vi "sitios sound.vi"() -> ()   [LabVIEW 2010]
uses:
  <vilib>/addons/PixeLINK/Low Level Functions/CAMERA_FEATURES.llb/TDPU-CameraFeatures-PixelFormat.ctl
  <vilib>/sound2/lvsound2.llb/Sound Data Format.ctl
  <vilib>/sound2/lvsound2.llb/Sound Output Task ID.ctl
  <vilib>/Utility/error.llb/DialogType.ctl
  <vilib>/Utility/file.llb/Write To Spreadsheet File (DBL).vi
  <vilib>/vision/NI_Vision_Development_Module.lvlib
panel:
  in  "Paso inicial":dbl=0.25
  out "Numeric":dbl
  out "output string":string
  in  "Sound Controls":T2={"device ID"=0, "sound format"={"sample rate (S/s)"=44000.0, "number of channels"=2, "bits per sample"=16}, "time (ms)"=200.0}
  in  "tiempo de espera (ms)":u32=5000
  out "Paso actual":i32
  in  "nombre archivo":string="paso"
  in  "Cantidad de pasos":u32=16
  in  "base path":path=path "C:/Users/veloz/Documents/tesis/codigos/Matlab/archivos"
  in  "Tamaño entre pasos":dbl=0.25
  out "Veces Realizado":i32
  in  "Veces":u16=1
  in  "Imagenes":i32=5
  in  "tiempo entre pasos (ms)":dbl=2000.0
  out "Tamaño del paso":dbl=4.0
  in  "Valor Inicial":dbl=-10.0
  out "Array":T3[](array[plugin-control])
  in  "Start":bool
  out "Image OUT":T3(plugin-control)
  out "new file path":path
  in  "stop":bool
  out "Imagenes tomadas":i32
  in  "Camara Parameters":T5 {"Pixel Format" items=["PIXEL_FORMAT_MONO8", "PIXEL_FORMAT_MONO16", "PIXEL_FORMAT_YUV422", "PIXEL_FORMAT_BAYER8_GRBG", "PIXEL_FORMAT_BAYER16_GRBG", "PIXEL_FORMAT_RGB24", "PIXEL_FORMAT_RGB48", "PIXEL_FORMAT_BAYER8_RGGB", "PIXEL_FORMAT_BAYER8_GBRG ", "PIXEL_FORMAT_BAYER8_BGGR ", "PIXEL_FORMAT_BAYER16_RGGB ", "PIXEL_FORMAT_BAYER16_GBRG", "PIXEL_FORMAT_BAYER16_BGGR", "PIXEL_FORMAT_RGB32"]}
  in  "Selector":u16(ring) items=["776002034"]
  in  "Streeam?":bool
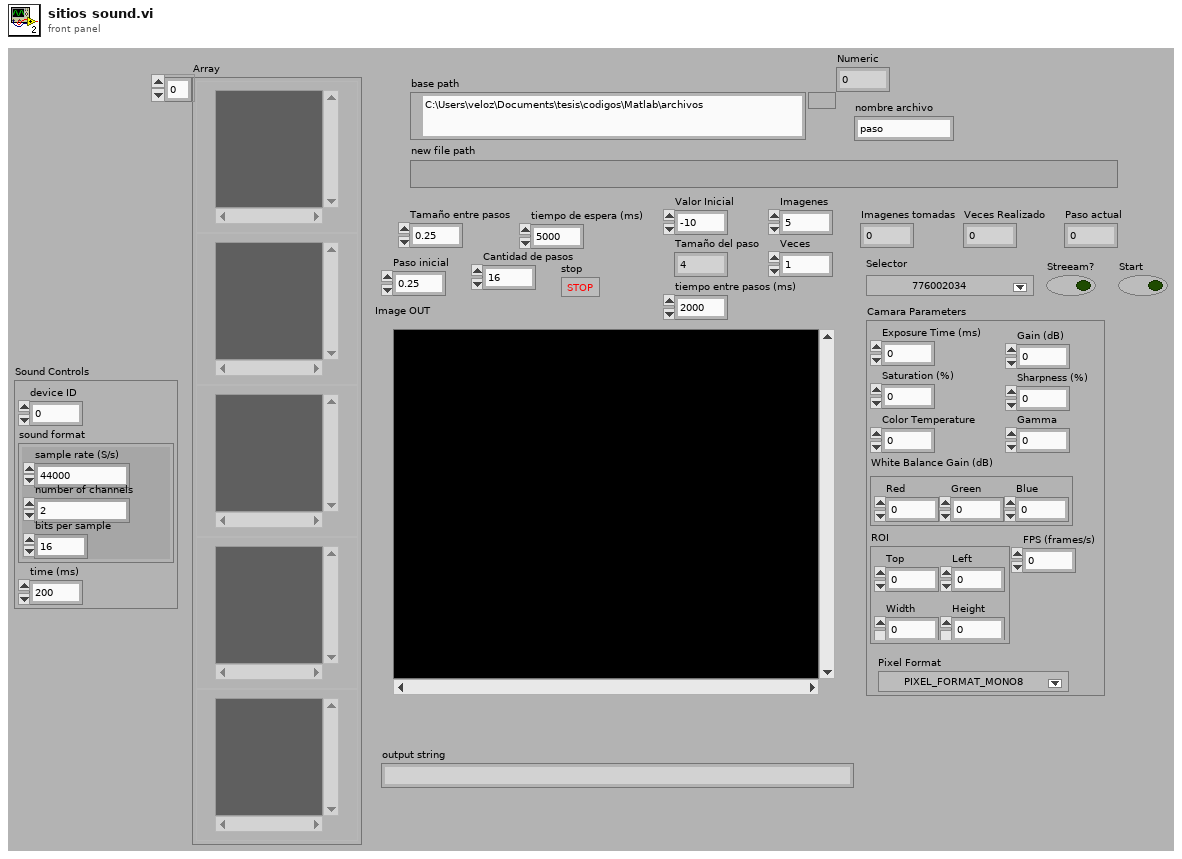
[diagram p1: front panel]
types:
  T1 = typedef "Sound Data Format.ctl" = cluster{"sample rate (S/s)":dbl, "number of channels":i32, "bits per sample":i32}
  T2 = cluster{"device ID":u32, "sound format":T1, "time (ms)":dbl}
  T3 = typedef "IMAQ Image.ctl" = refnum<image>
  T4 = typedef "TDPU-CameraFeatures-PixelFormat.ctl" = u16
  T5 = cluster{"Exposure Time (ms)":dbl, "Gain (dB)":dbl, "Saturation (%)":dbl, "Sharpness (%)":dbl, "Color Temperature":dbl, "ROI":cluster{"Top":i32, "Left":i32, "Width":i32, "Height":i32}, "White Balance Gain (dB)":cluster{"Red":dbl, "Green":dbl, "Blue":dbl}, "Gamma":dbl, "Pixel Format":T4, "FPS (frames/s)":i32}
  T6 = typedef "Sound Output Task ID.ctl" = u32
  T7 = cluster{"task ID":T6, "error":errorcluster, "sound format":T1}
  T8 = cluster{"hCamera":u32, "Error":errorcluster, "uSerialNumber OUT":u32}
  T9 = cluster{"hCamera":u32, "Error":errorcluster, "uSerialNumber":u32}
  T10 = typedef "Image Type" = u32
  T11 = typedef "DialogType.ctl" = u16
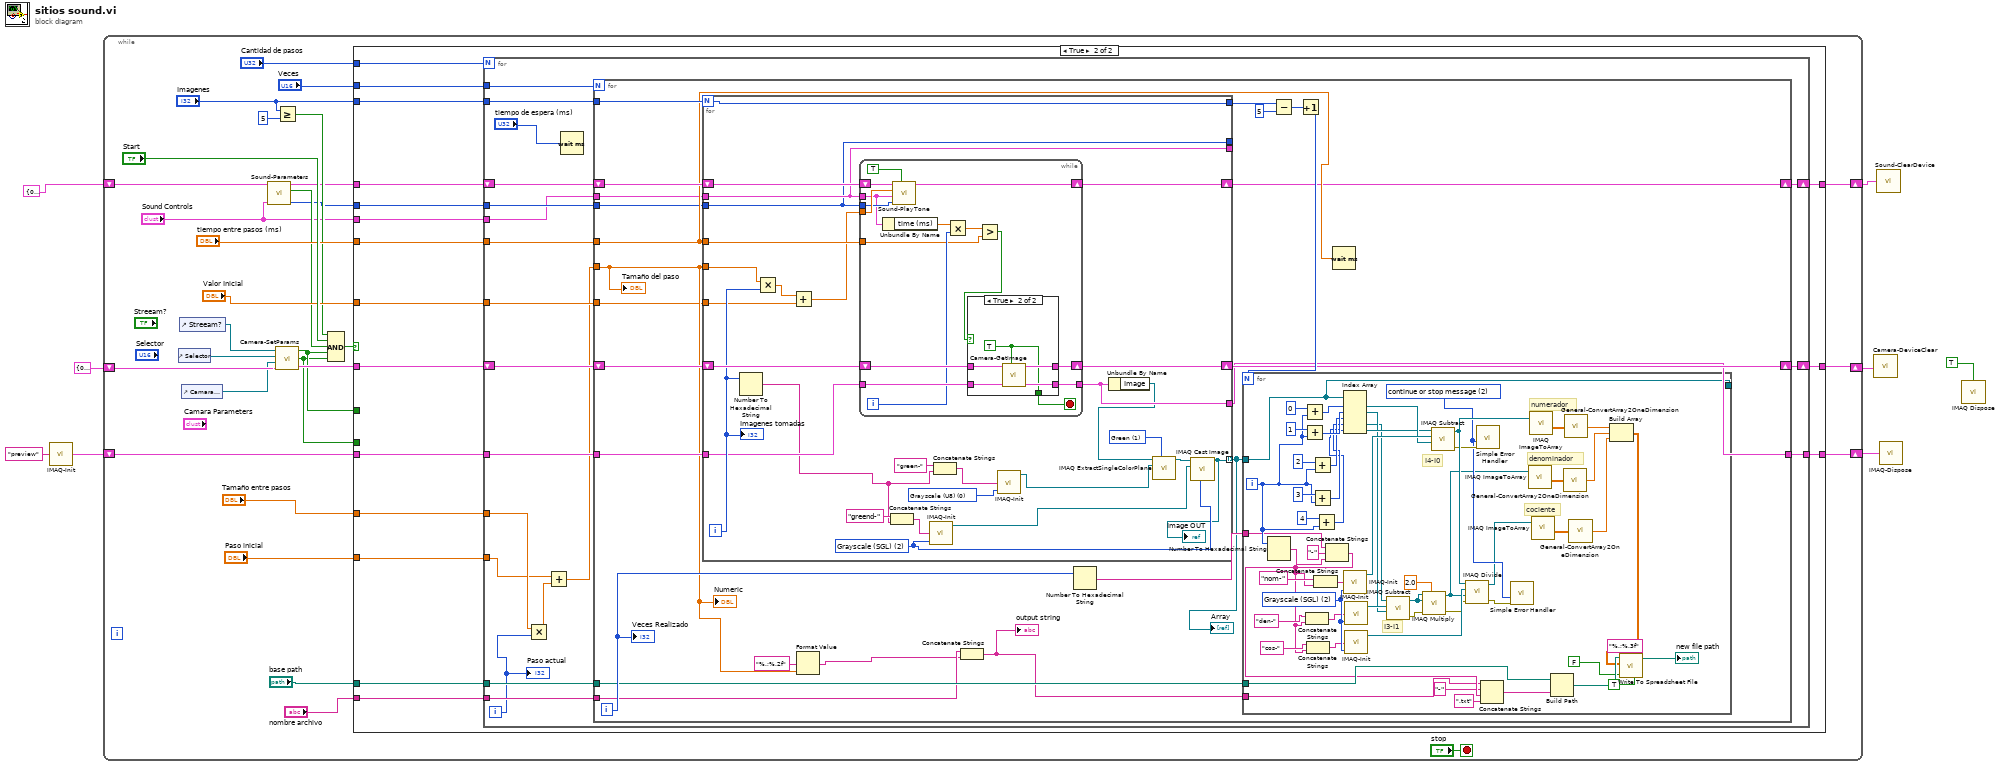
[diagram p0: block diagram]
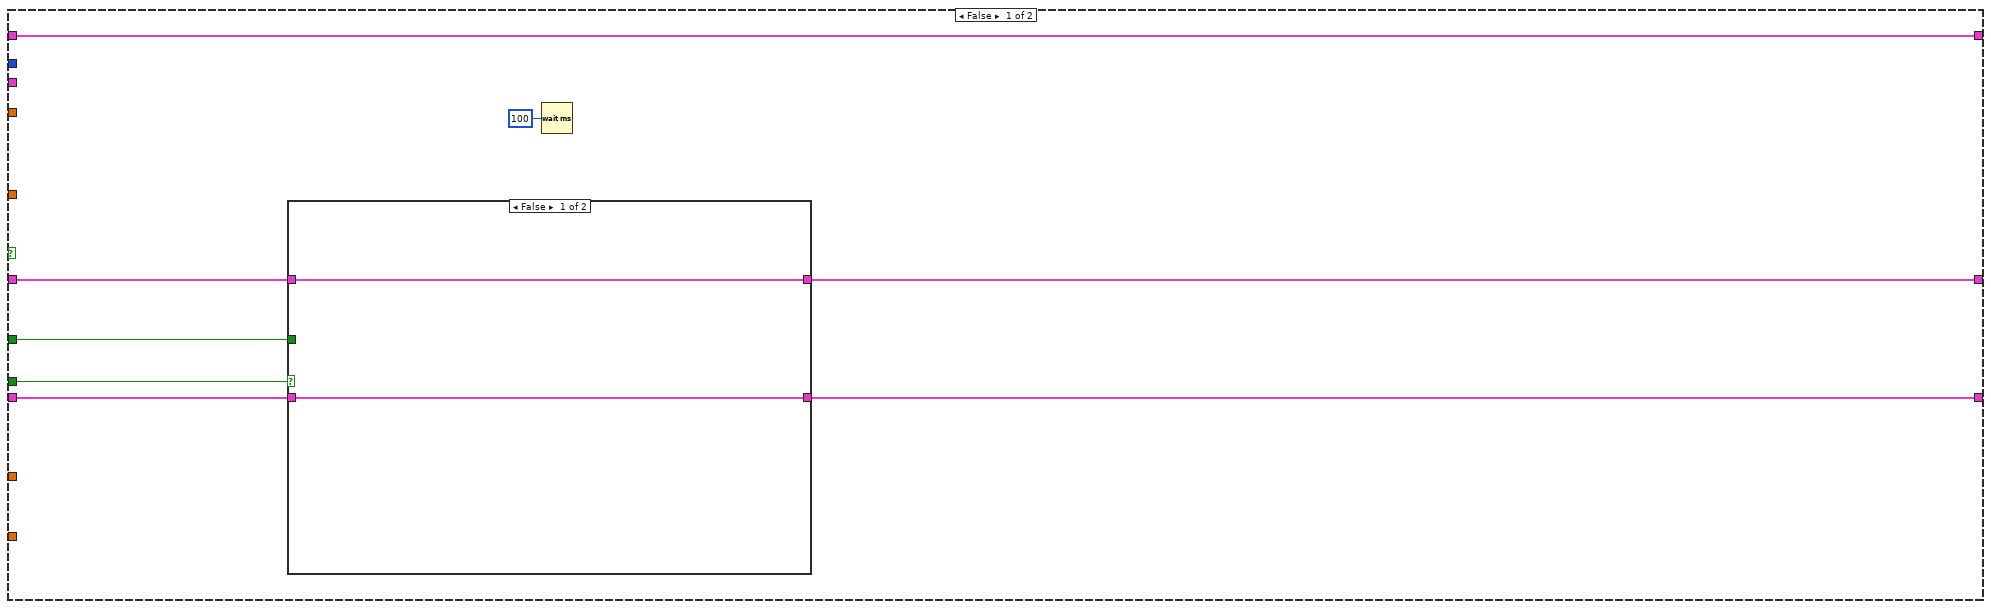
[diagram p2: hidden frame]
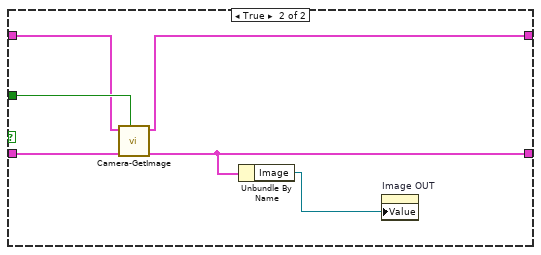
[diagram p3: hidden frame]
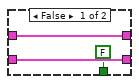
[diagram p4: hidden frame]
diagram:
  n1 = call "IMAQ-Init.vi"("Image Name"="preview") -> ("Image Device OUT"=w5:cluster{"Image":T3, "errorImage":errorcluster})  [unwired: 2 in, 2 out]
  n2 = while {
    shift-right: [w30] -> w3
    shift-left: T8 {"hCamera"=0, "Error"={"status"=FALSE, "code"=0, "source"=""}, "uSerialNumber OUT"=0} ("Camera Device  IN") -> [w34]
    shift-right: [w31] -> w1
    shift-left: T7 {"task ID"=0, "error"={"status"=TRUE, "code"=0, "source"=""}, "sound format"={"sample rate (S/s)"=0.0, "number of channels"=0, "bits per sample"=0}} ("Sound Device OUT") -> [w14]
    shift-right: [w18] -> w4
    shift-left: w5 -> [w20]
    stop <- "stop" stop-if-true
    n3 = control-ref of="Selector"() -> (w38:refnum<vi>)
    n4 = control-ref of="Streeam?"() -> (w37:refnum<vi>)
    n5 = control-ref of="Camara Parameters"() -> (w36:refnum<vi>)
    n6 = call "Sound-Parameters.vi"("Sound Controls"="Sound Controls", "Sound Device IN"=w14) -> ("#samples"=w11:u32, "En funcionamiento?"=w12:bool, "Sound Device OUT"=w13:T7)  [unwired: 3 in]
    n7 = call "Camera-SetParams.vi"("Camera Device  IN"=w34, "Camera Parameters"=w36, "Selector"=w38, "Stream?"=w37) -> ("Camera Device OUT"=w35:T9, "Funciona?"=w17:bool, "Stream? OUT"=w19:bool)
    n8 = Greater Or Equal?(x="Imagenes", y=5) -> (x >= y?=w25:bool)
    n9 = Compound Arithmetic op=AND(w25, "Start", w12, w19, w17) -> (w33:bool)
    n10 = case shown="True" w33 {
      tunnel: w35 -> [w42 w71]
      tunnel: [w41 w66] -> w30
      tunnel: w13 -> [w45 w58]
      tunnel: [w45 w70] -> w31
      tunnel: "tiempo entre pasos (ms)" -> [_ w68]
      tunnel: "Imagenes" -> [_ w69]
      tunnel: "Valor Inicial" -> [_ w67]
      tunnel: "Veces" -> [_ w65]
      tunnel: "base path" -> [_ w64]
      tunnel: "nombre archivo" -> [_ w63]
      tunnel: w20 -> [w44 w62]
      tunnel: w19 -> [w43 _]
      tunnel: [w40 w61] -> w18
      tunnel: w17 -> [w39 _]
      tunnel: "Tamaño entre pasos" -> [_ w60]
      tunnel: "Cantidad de pasos" -> [_ w59]
      tunnel: w11 -> [_ w57]
      tunnel: "Sound Controls" -> [_ w56]
      tunnel: "Paso inicial" -> [_ w55]
      frame False {
        n11 = case shown="False" w39 {
          tunnel: w44 -> [w47 w54]
          tunnel: w43 -> [_ w53]
          tunnel: w42 -> [w48 w52]
          tunnel: [w48 w51] -> w41
          tunnel: [w47 w50] -> w40
          frame False {
          }
          frame True {
            n12 = call "Camera-GetImage.vi"("Streeam"=w53, "Image Device IN"=w54, "Camera Device IN"=w52) -> ("Image Device OUT"=w50:cluster{"Image":T3, "errorImage":errorcluster}, "Camera Device OUT"=w51:T9)  [unwired: 4 in]
            n13 = Unbundle By Name(w50) -> ("Image"=w49:T3)
            n14 = property on="Image OUT" class="ImageControl"("Value"=w49) -> ()  [unwired: 2 in, 2 out]
          }
        }
        n15 = Wait (ms)(milliseconds to wait=u32 100) -> ()  [unwired: 1 out]
      }
      frame True {
        n16 = for {
          N: w59 -> [_]
          tunnel: w69 -> [w89]
          tunnel: w68 -> [w88]
          tunnel: w67 -> [w87]
          tunnel: w65 -> [w84]
          tunnel: w64 -> [w83]
          tunnel: w63 -> [w82]
          tunnel: w62 -> [w81]
          tunnel: [w80] -> w61
          shift-right: [w85] -> w66
          shift-left: w71 -> [w91]
          shift-right: [w90] -> w70
          shift-left: w58 -> [w86]
          tunnel: w60 -> [w79]
          tunnel: w57 -> [w77]
          tunnel: w56 -> [w76]
          tunnel: w55 -> [w75]
          i -> [w74]
          n17 = Multiply(x=w79, y=w74) -> (x*y=w73:dbl)
          n18 = Add(x=w75, y=w73) -> (x+y=w72:dbl)
          n19 = Wait (ms)(milliseconds to wait="tiempo de espera (ms)") -> ()  [unwired: 1 out]
          n20 = for {
            N: w84 -> [_]
            tunnel: w89 -> [w114]
            tunnel: w88 -> [w96]
            tunnel: w72 -> [w100]
            tunnel: w87 -> [w97]
            shift-right: [w93] -> w90
            shift-left: w86 -> [w108]
            shift-right: [w107] -> w85
            shift-left: w91 -> [w115]
            tunnel: w83 -> [w105]
            tunnel: w82 -> [w101]
            tunnel: w81 -> [w104]
            tunnel: [w103] -> w80
            tunnel: w77 -> [w95]
            tunnel: w76 -> [w94]
            i -> [w106]
            n21 = for {
              N: w114 -> [w189]
              tunnel: w96 -> [w196]
              tunnel: w100 -> [w194]
              tunnel: w97 -> [w192]
              tunnel: [w175] -> w102 mode=indexing
              tunnel: [w189] -> w113
              shift-right: [w199] -> w93
              shift-left: w108 -> [w200]
              shift-right: [w197] -> w107
              shift-left: w115 -> [w198]
              tunnel: w104 -> [w186]
              tunnel: [w185] -> w103
              tunnel: w95 -> [w173]
              tunnel: w94 -> [w174]
              tunnel: [w174] -> _
              tunnel: [w173] -> _
              i -> [w195]
              w180 = T10 2 items=["Grayscale (U8)", "Grayscale (I16)", "Grayscale (SGL)", "Complex (CSG)", "RGB (U32)", "HSL (U32)", "RGB (U64)", "Grayscale (U16)"] ("Image Type")
              w184 = 1 items=["Red", "Green", "Blue", "Hue", "Saturation", "Luminance", "Value", "Intensity"] ("Color Plane")
              w187 = T10 0 items=["Grayscale (U8)", "Grayscale (I16)", "Grayscale (SGL)", "Complex (CSG)", "RGB (U32)", "HSL (U32)", "RGB (U64)", "Grayscale (U16)"] ("Image Type")
              n22 = Number To Hexadecimal String(2:w195) -> (0:w178:string)  [unwired: 1 in]
              n23 = Multiply(x=w194, y=w195) -> (x*y=w191:dbl)
              n24 = Add(x=w191, y=w192) -> (x+y=w193:dbl)
              n25 = while {
                tunnel: w196 -> [w203]
                tunnel: w193 -> [w212]
                tunnel: w186 -> [w211]
                tunnel: [w210] -> w185
                tunnel: w174 -> [w207]
                tunnel: w173 -> [w209]
                shift-right: [w213] -> w197
                shift-left: w198 -> [w214]
                shift-right: [w215] -> w199
                shift-left: w200 -> [w216]
                i -> [w205]
                stop <- w202 stop-if-true
                n26 = Unbundle By Name(w207) -> ("time (ms)"=w206:dbl)
                n27 = call "Sound-PlayTone.vi"("sound?"=TRUE ("DAQ?"), "# samples"=w209, "Sound Controls"=w207, "Frecuencia"=w212, "Sound Device IN"=w216) -> ("Sound Device OUT"=w215:T7)  [unwired: 3 in, 1 out]
                n28 = Multiply(x=w206, y=w205) -> (x*y=w204:dbl)
                n29 = Greater?(x=w204, y=w203) -> (0:w201:bool)
                n30 = case shown="True" w201 {
                  tunnel: w214 -> [w219 w224]
                  tunnel: [w219 w223] -> w213
                  tunnel: w211 -> [w218 w222]
                  tunnel: [w218 w221] -> w210
                  tunnel: [FALSE ("Streeam") w220] -> w202
                  frame False {
                  }
                  frame True {
                    w220 = TRUE ("Streeam")
                    n31 = call "Camera-GetImage.vi"("Streeam"=w220, "Image Device IN"=w222, "Camera Device IN"=w224) -> ("Image Device OUT"=w221:cluster{"Image":T3, "errorImage":errorcluster}, "Camera Device OUT"=w223:T9)  [unwired: 4 in]
                  }
                }
              }
              n32 = Concatenate Strings("greend-" ("string"), w178) -> (w177:string)
              n33 = call "IMAQ-Init.vi"("Image Type"=w180, "Image Name"=w177) -> ("Image OUT"=w181:T3)  [unwired: 1 in, 2 out]
              n34 = Concatenate Strings("green-" ("string"), w178) -> (w188:string)
              n35 = call "IMAQ-Init.vi"("Image Type"=w187, "Image Name"=w188) -> ("Image OUT"=w183:T3)  [unwired: 1 in, 2 out]
              n36 = Unbundle By Name(w185) -> ("Image"=w176:T3)
              n37 = call "IMAQ ExtractSingleColorPlane"("Color Plane"=w184, "Image Dst"=w183, "Image Src"=w176) -> ("Image Dst Out"=w182:T3)  [unwired: 7 in, 1 out]
              n38 = call "IMAQ Cast Image"("Image Type"=w180, "Image Dst"=w181, "Image Src"=w182) -> ("Image Dst Out"=w175:T3)  [unwired: 7 in, 1 out]
              "Image OUT" <- w175
              "Imagenes tomadas" <- w195
            }
            "Array" <- w102
            n39 = Format Value(format string="%.;%.2f", value (0)=w100) -> (output string=w98:string)  [unwired: 1 in]
            n40 = Concatenate Strings(w101, w98) -> (w92:string)
            "output string" <- w92
            n41 = Number To Hexadecimal String(2:w106) -> (0:w109:string)  [unwired: 1 in]
            n42 = Subtract(x=w113, y=5) -> (x-y=w111:i32)
            n43 = Increment(x=w111) -> (x+1=w110:i32)
            n44 = for {
              N: w110 -> [_]
              tunnel: w102 -> [w154]
              tunnel: [w154] -> _
              tunnel: w109 -> [w150]
              tunnel: w105 -> [w147]
              tunnel: w92 -> [w138]
              i -> [w153]
              w128 = T11 2 items=["no dialog", "OK message", "continue or stop message", "OK message + warnings", "continue/stop + warnings"] ("type of dialog (OK msg:1)")
              w137 = T10 2 items=["Grayscale (U8)", "Grayscale (I16)", "Grayscale (SGL)", "Complex (CSG)", "RGB (U32)", "HSL (U32)", "RGB (U64)", "Grayscale (U16)"] ("Image Type")
              # "I3-I1"
              # "I4-I0"
              # "cociente"
              # "denominador"
              # "numerador"
              n45 = Number To Hexadecimal String(2:w153) -> (0:w151:string)  [unwired: 1 in]
              n46 = Add(x=0, y=w153) -> (x+y=w163:i32)
              n47 = Add(x=1, y=w153) -> (x+y=w162:i32)
              n48 = Add(x=2, y=w153) -> (x+y=w161:i32)
              n49 = Add(x=3, y=w153) -> (x+y=w160:i32)
              n50 = Add(x=4, y=w153) -> (x+y=w159:i32)
              n51 = Concatenate Strings(w150, "-" ("string"), w151) -> (w145:string)
              n52 = Concatenate Strings("den-" ("Image Name"), w145) -> (w118:string)
              n53 = Concatenate Strings("cos-" ("Image Name"), w145) -> (w117:string)
              n54 = Concatenate Strings("nom-" ("Image Name"), w145) -> (w167:string)
              n55 = Index Array(array=w154, index #1=w163, index #2=w162, index #3=w161, index #4=w160, index #5=w159) -> (element #1=w136:T3, element #2=w134:T3, element #4=w133:T3, element #5=w135:T3)  [unwired: 1 out]
              n56 = call "IMAQ-Init.vi"("Image Type"=w137, "Image Name"=w167) -> ("Image OUT"=w155:T3)  [unwired: 1 in, 2 out]
              n57 = call "IMAQ-Init.vi"("Image Type"=w137, "Image Name"=w118) -> ("Image OUT"=w157:T3)  [unwired: 1 in, 2 out]
              n58 = call "IMAQ-Init.vi"("Image Type"=w137, "Image Name"=w117) -> ("Image OUT"=w148:T3)  [unwired: 1 in, 2 out]
              n59 = call "IMAQ Subtract"("Image Src A"=w133, "Image Dst"=w157, "Image Src B"=w134) -> ("Image Dst Out"=w156:T3, "error out"=w132:errorcluster)  [unwired: 4 in]
              n60 = call "IMAQ Multiply"("Image Src A"=w156, "Constant"=sgl 2.0, "Image Dst"=w156, "error in (no error)"=w132) -> ("Image Dst Out"=w125:T3, "error out"=w131:errorcluster)  [unwired: 3 in]
              n61 = call "IMAQ Subtract"("Image Src A"=w135, "Image Dst"=w155, "Image Src B"=w136) -> ("Image Dst Out"=w149:T3, "error out"=w129:errorcluster)  [unwired: 4 in]
              n62 = call "IMAQ Divide"("Image Src A"=w149, "Image Dst"=w148, "Image Src B"=w125, "error in (no error)"=w131) -> ("Image Dst Out"=w126:T3, "error out"=w130:errorcluster)  [unwired: 3 in]
              n63 = call <vilib>:"Simple Error Handler.vi"("type of dialog (OK msg:1)"=w128, "error in (no error)"=w129) -> ()  [unwired: 3 in, 5 out]
              n64 = Concatenate Strings(w138, "-" ("string"), w145, ".txt" ("string")) -> (w146:string)
              n65 = call <vilib>:"Simple Error Handler.vi"("type of dialog (OK msg:1)"=w128, "error in (no error)"=w130) -> ()  [unwired: 3 in, 5 out]
              n66 = call "IMAQ ImageToArray"("Image"=w125) -> ("Image Pixels (Float)"=w122:sgl[][])  [unwired: 3 in, 4 out]
              n67 = call "IMAQ ImageToArray"("Image"=w149) -> ("Image Pixels (Float)"=w124:sgl[][])  [unwired: 3 in, 4 out]
              n68 = call "IMAQ ImageToArray"("Image"=w126) -> ("Image Pixels (Float)"=w121:sgl[][])  [unwired: 3 in, 4 out]
              n69 = Build Path(base path=w147, name or relative path=w146) -> (appended path=w144:path)
              n70 = call "General-ConvertArray2OneDimension.vi"("Input Array"=w122) -> ("Output Array"=w120:dbl[])
              n71 = call "General-ConvertArray2OneDimension.vi"("Input Array"=w124) -> ("Output Array"=w123:dbl[])
              n72 = call "General-ConvertArray2OneDimension.vi"("Input Array"=w121) -> ("Output Array"=w119:dbl[])
              n73 = Build Array(w123, w120, w119) -> (w143:dbl[][])
              n74 = call-poly <vilib>:"Write To Spreadsheet File.vi"("transpose? (no:F)"=TRUE, "format (%.3f)"="%.;%.3f", "append to file? (new file:F)"=FALSE, "2D data"=w143, "file path (dialog if empty)"=w144) -> ("new file path (Not A Path if cancelled)"=→"new file path":path)  [unwired: 3 in]
            }
            n75 = Wait (ms)(milliseconds to wait=w96) -> ()  [unwired: 1 out]
            "Veces Realizado" <- w106
            "Tamaño del paso" <- w100
            "Numeric" <- w100
          }
          "Paso actual" <- w74
        }
      }
    }
  }
  n76 = call "Camera-DeviceClear.vi"("Camera Device OUT"=w3) -> ()
  n77 = call "Sound-ClearDevice.vi"("Sound Device OUT"=w1) -> ()
  n78 = call "IMAQ-Dispose.vi"("Image Device IN"=w4) -> ()
  n79 = call "IMAQ Dispose"("All Images? (No)"=TRUE) -> ()  [unwired: 5 in, 1 out]
